vi "sCMOS_define_ROI.vi"(1 "Global Rectangle":i32[](array[numeric])) -> (0 "ROI cluster":T1)   [LabVIEW 2015]
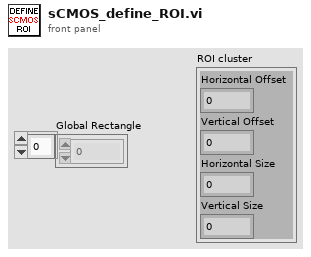
[diagram p1: front panel]
types:
  T1 = cluster{"Horizontal Offset":i32, "Vertical Offset":i32, "Horizontal Size":i32, "Vertical Size":i32}
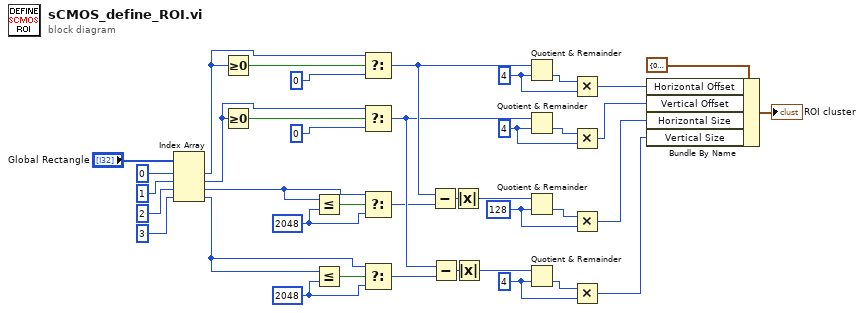
[diagram p0: block diagram]
diagram:
  w19 = 2048 ("y")
  w20 = 2048 ("y")
  w2 = 4 ("y")
  w5 = 128 ("y")
  w8 = 4 ("y")
  w11 = 4 ("y")
  n1 = Index Array(array="Global Rectangle", index #1=0 ("index"), index #2=1 ("index"), index #3=2 ("index"), index #4=3 ("index")) -> (element #1=w26:i32, element #2=w24:i32, element #3=w21:i32, element #4=w17:i32)
  n2 = Greater Or Equal To 0?(x=w26) -> (x >= 0?=w30:bool)
  n3 = Greater Or Equal To 0?(x=w24) -> (x >= 0?=w27:bool)
  n4 = Less Or Equal?(x=w21, y=w20) -> (x <= y?=w22:bool)
  n5 = Less Or Equal?(x=w17, y=w19) -> (x <= y?=w18:bool)
  n6 = Select(t=w26, s=w30, f=0) -> (s? t:f=w25:i32)
  n7 = Select(t=w24, s=w27, f=0) -> (s? t:f=w23:i32)
  n8 = Select(t=w21, s=w22, f=w20) -> (s? t:f=w16:i32)
  n9 = Select(t=w17, s=w18, f=w19) -> (s? t:f=w15:i32)
  n10 = Subtract(x=w25, y=w16) -> (x-y=w31:i32)
  n11 = Subtract(x=w23, y=w15) -> (x-y=w32:i32)
  n12 = Absolute Value(x=w31) -> (abs(x)=w34:i32)
  n13 = Absolute Value(x=w32) -> (abs(x)=w33:i32)
  n14 = Quotient & Remainder(x=w25, y=w11) -> (floor(x/y)=w12:i32)  [unwired: 1 out]
  n15 = Quotient & Remainder(x=w23, y=w8) -> (floor(x/y)=w9:i32)  [unwired: 1 out]
  n16 = Quotient & Remainder(x=w34, y=w5) -> (floor(x/y)=w6:i32)  [unwired: 1 out]
  n17 = Quotient & Remainder(x=w33, y=w2) -> (floor(x/y)=w3:i32)  [unwired: 1 out]
  n18 = Multiply(x=w12, y=w11) -> (x*y=w10:i32)
  n19 = Multiply(x=w9, y=w8) -> (x*y=w7:i32)
  n20 = Multiply(x=w6, y=w5) -> (x*y=w4:i32)
  n21 = Multiply(x=w3, y=w2) -> (x*y=w1:i32)
  n22 = Bundle By Name(cluster=T1 {"Horizontal Offset"=0, "Vertical Offset"=0, "Horizontal Size"=0, "Vertical Size"=0} ("Sub Region"), "Horizontal Offset"=w10, "Vertical Offset"=w7, "Horizontal Size"=w4, "Vertical Size"=w1) -> (→"ROI cluster":T1)
